vi "Configure SRE.vi"(8 "error in (no error)":errorcluster, 9 "Service Request Enable Register (0)":u8, 11 "VISA resource name":refnum<visa-resource-name>) -> (0 "error out":errorcluster, 3 "VISA resource name out":refnum<visa-resource-name>)   [LabVIEW 2010, in "Temptronic TP04300.lvlib"]
doc: "This VI configures <b>*SRE</b> Service Request Enable (mask) Register.\n\nValid Range: 0 - 255\nDefault: 0"
uses:
  Temptronic TP04300.lvlib
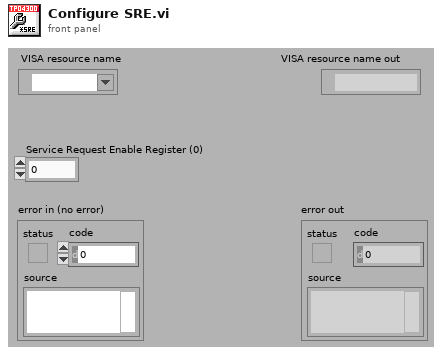
[diagram p1: front panel]
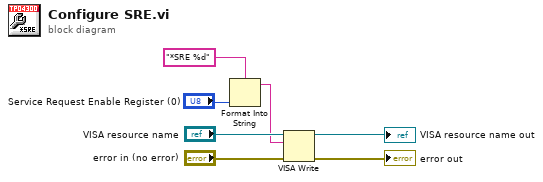
[diagram p0: block diagram]
diagram:
  n1 = Format Into String(format string="*SRE %d", "Service Request Enable Register (0)") -> (resulting string=w5:string)  [unwired: 2 in, 1 out]
  n2 = VISA Write(VISA resource name="VISA resource name", write buffer=w5, error in (no error)="error in (no error)") -> (VISA resource name out=→"VISA resource name out":refnum<visa-resource-name>, error out=→"error out":errorcluster)  [unwired: 1 out]
